vi "DSF.Execution.Runtime.Plugin Manager.Load Plugin.vi"(8 "error in (no error)":errorcluster, 10 "Plugin name":string, 11 "Plugin Manager in":refnum<class "Plugin Manager.lvclass">) -> (0 "error out":errorcluster, 2 "Plugin Classes":T1, 3 "Plugin Manager out":refnum<class "Plugin Manager.lvclass">)   [LabVIEW 2016, in "DSF.Engine.lvlib" / "Plugin Manager.lvclass"]
uses:
  Plugin Manager.lvclass
  Shared/Classes/Plugin/DSF.Shared.Configuration.Plugin.lvclass
  Shared/Classes/Transfer Group/DSF.Shared.Configuration.Transfer Group.lvclass
  Shared/Classes/Transfer/DSF.Shared.Configuration.Transfer.lvclass
  Shared/Typedefs/DSF.Shared.Typedefs.Plugin Classes.Configuration.ctl
  DSF.Shared.lvlib
  Plugin/DSF.Engine.Runtime.Plugin.lvclass
  Shared/Typedefs/DSF.Shared.Typedefs.Plugin Classes.Runtime.ctl
  Shared/Typedefs/DSF.Shared.Typedefs.Plugin Classes.ctl
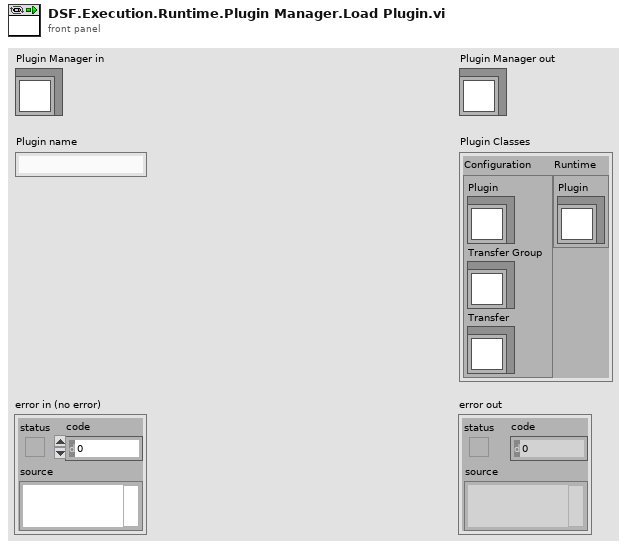
[diagram p1: front panel]
types:
  T1 = typedef "DSF.Shared.lvlib/DSF.Shared.Typedefs.Plugin Classes.ctl" = cluster{"Configuration":T2, "Runtime":T3}
  T2 = typedef "DSF.Shared.lvlib/DSF.Shared.Typedefs.Plugin Classes.Configuration.ctl" = cluster{"Plugin":refnum<class "DSF.Shared.Configuration.Plugin.lvclass">, "Transfer Group":refnum<class "DSF.Shared.Configuration.Transfer Group.lvclass">, "Transfer":refnum<class "DSF.Shared.Configuration.Transfer.lvclass">}
  T3 = typedef "DSF.Shared.lvlib/DSF.Shared.Typedefs.Plugin Classes.Runtime.ctl" = cluster{"Plugin":refnum<class "DSF.Engine.Runtime.Plugin.lvclass">}
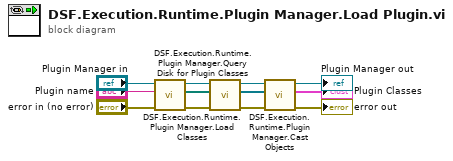
[diagram p0: block diagram]
diagram:
  n1 = call "DSF.Execution.Runtime.Plugin Manager.Query Disk for Plugin Classes.vi"("error in (no error)"="error in (no error)", "Plugin name"="Plugin name", "Plugin Manager in"="Plugin Manager in") -> ("error out"=w7:errorcluster, "Plugin class paths"=w9:path[], "Plugin Manager out"=w8:refnum<class "Plugin Manager.lvclass">)  [unwired: 6 in]
  n2 = call "DSF.Execution.Runtime.Plugin Manager.Load Classes.vi"("error in (no error)"=w7, "class paths"=w9, "Plugin Manager in"=w8) -> ("error out"=w4:errorcluster, "objects"=w6:refnum<class>[], "Plugin Manager out"=w5:refnum<class "Plugin Manager.lvclass">)  [unwired: 6 in]
  n3 = call "DSF.Execution.Runtime.Plugin Manager.Cast Objects.vi"("error in (no error)"=w4, "Plugin objects"=w6, "Plugin Manager in"=w5) -> ("error out"=→"error out":errorcluster, "Plugin Classes"=→"Plugin Classes":T1, "Plugin Manager out"=→"Plugin Manager out":refnum<class "Plugin Manager.lvclass">)  [unwired: 6 in]
